vi "CLSUIP_ShouldReplaceControl.vi"(4 "error in (no error)":errorcluster, 5 "Terminal Index":u32, 6 "ConPane":refnum<vi>, 7 "VIRetooler":refnum<class "VIRetooler.lvclass">) -> (0 "error out":errorcluster, 1 "Should replace?":bool, 3 "VIRetooler 2":refnum<class "VIRetooler.lvclass">)   [LabVIEW 2021, in "MemberVICreation.lvlib" / "VIRetooler.lvclass"]
uses:
  <resource>/Framework/Providers/LVClassLibrary/NewAccessors/VIRetooler/VIRetooler.lvclass
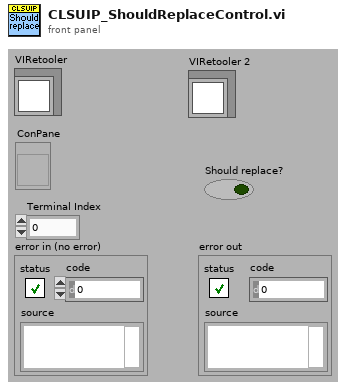
[diagram p1: front panel]
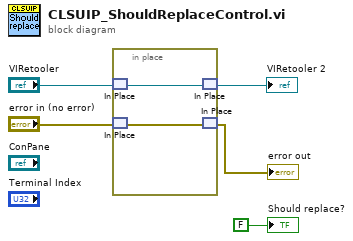
[diagram p0: block diagram]
diagram:
  n1 = in-place {
    n2 = in-place-match #1("VIRetooler") -> (w7:refnum<class "VIRetooler.lvclass">)
    n3 = in-place-match #2("error in (no error)") -> (w6:errorcluster)
    n4 = in-place-match #1(w7) -> (→"VIRetooler 2":refnum<class "VIRetooler.lvclass">)
    n5 = in-place-match #2(w6) -> (→"error out":errorcluster)
  }
  "Should replace?" <- FALSE ("Is Dynamic?")
